vi "Retrieve.vi"   [LabVIEW 2026, in "synnax_lib.lvlib" / "Synnax Client.lvclass"]
uses:
  Synnax Client.lvclass
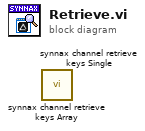
[diagram p0: block diagram]
diagram:
  n1 = call "synnax channel retrieve keys Array.vi"() -> ()  [unwired: 11 in, 5 out]
  n2 = call "synnax channel retrieve keys Single.vi"() -> ()  [unwired: 11 in, 5 out]
